vi "数据上传Z070A.vi"(1 "数据数组":string[](array[string]), 2 "合格Z030":bool, 3 "操作者":string, 4 "产品ID":string) -> ()   [LabVIEW 2011]
uses:
  <vilib>/Utility/error.llb/whitespace.ctl
panel:
  in  "error in (no error)":errorcluster
  out "error out":errorcluster
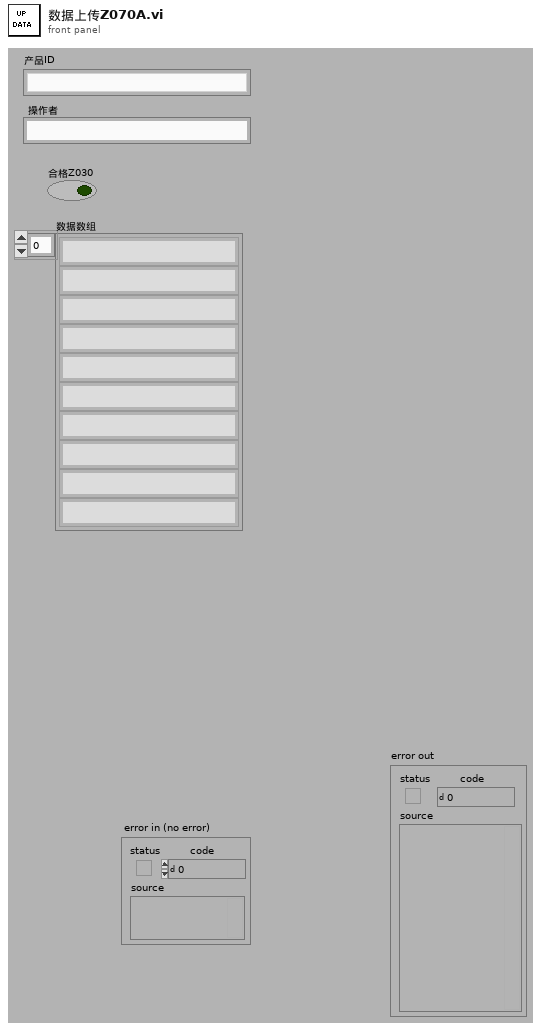
[diagram p1: front panel]
types:
  T1 = typedef "whitespace.ctl" = u16
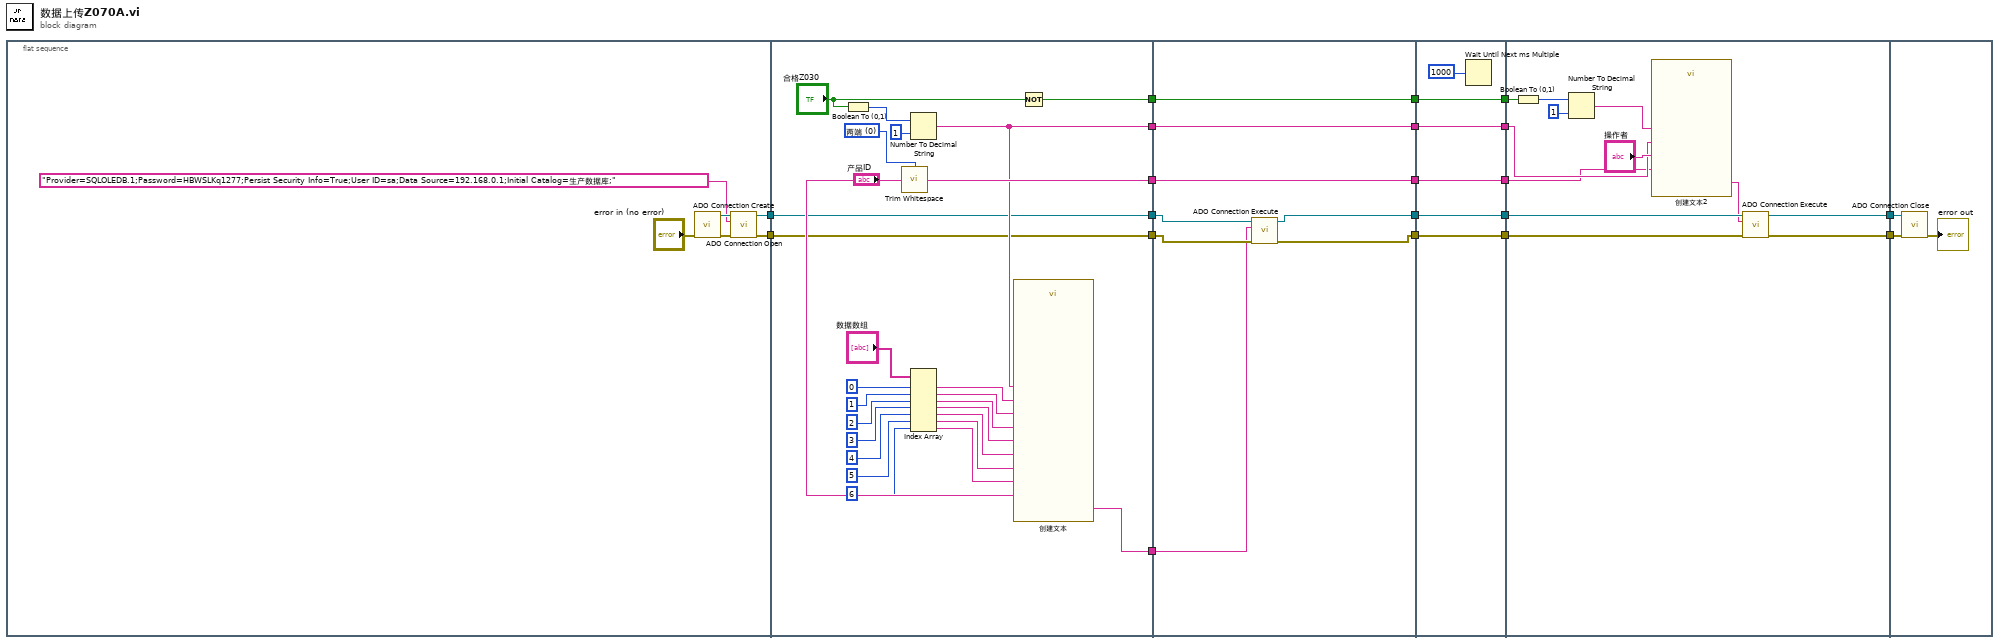
[diagram p0: block diagram]
diagram:
  n1 = flat-sequence {
    tunnel: [w22] -> w20
    tunnel: [w23] -> w19
    tunnel: w20 -> [w27]
    tunnel: w19 -> [w28]
    tunnel: [w28] -> w11
    tunnel: [w27] -> w9
    tunnel: [w43] -> w7
    tunnel: [w44] -> w5
    tunnel: [w46] -> w3
    tunnel: [w29] -> w1
    tunnel: w11 -> [w57]
    tunnel: [w56] -> w10
    tunnel: w9 -> [w55]
    tunnel: [w54] -> w8
    tunnel: w7 -> [w60]
    tunnel: [w60] -> w6
    tunnel: w5 -> [w59]
    tunnel: [w59] -> w4
    tunnel: w3 -> [w58]
    tunnel: [w58] -> w2
    tunnel: w1 -> [w53]
    tunnel: w10 -> [w66]
    tunnel: [w66] -> w18
    tunnel: w8 -> [w65]
    tunnel: [w65] -> w17
    tunnel: w6 -> [w64]
    tunnel: [w64] -> w16
    tunnel: w4 -> [w63]
    tunnel: [w63] -> w15
    tunnel: [w61] -> w12
    tunnel: w2 -> [w61]
    tunnel: w18 -> [w72]
    tunnel: w17 -> [w71]
    tunnel: w16 -> [w74]
    tunnel: w15 -> [w73]
    tunnel: [w69] -> w14
    tunnel: [w68] -> w13
    tunnel: w12 -> [w67]
    tunnel: w14 -> [w80]
    tunnel: w13 -> [w79]
    frame #0 {
      n2 = call "ADO Connection Create.vi"("error in (no error)"="error in (no error)") -> ("error out"=w25:errorcluster, "ADODB._Connection Out"=w24:refnum<k7>)  [unwired: 9 out]
      n3 = call "ADO Connection Open.vi"("error in (no error)"=w25, "ConnectionString"="Provider=SQLOLEDB.1;Password=HBWSLKq1277;Persist Security Info=True;User ID=sa;Data Source=192.168.0.1;Initial Catalog=生产数据库;" ("字符串 2"), "ADODB._Connection In"=w24) -> ("error out"=w22:errorcluster, "ADODB._Connection Out"=w23:refnum<k7>)  [unwired: 7 out]
    }
    frame #1 {
      w52 = T1 0 items=["两端", "字符串首端", "字符串末端"] ("location (both)")
      n4 = Boolean To (0,1)(Boolean="合格Z030") -> (0, 1=w51:i16)
      n5 = call <vilib>:"Trim Whitespace.vi"("string"="产品ID", "location (both)"=w52) -> ("trimmed string"=w44:string)
      n6 = Number To Decimal String(number=w51, width (-)=i16 1 ("宽度(-)")) -> (decimal integer string=w43:string)
      n7 = Index Array(array="数据数组", index #1=0 ("索引"), index #2=1 ("索引"), index #3=2 ("索引"), index #4=3 ("索引"), index #5=4 ("索引"), index #6=5 ("索引"), index #7=6 ("索引")) -> (element #1=w42:string, element #2=w41:string, element #3=w40:string, element #4=w39:string, element #5=w38:string, element #6=w37:string, element #7=w36:string)
      n8 = call "创建文本"("合格"=w43, "左空载峰值扭矩"=w42, "左空载平均扭矩"=w41, "左空载扭差"=w40, "右空载峰值扭矩"=w39, "右空载平均扭矩"=w38, "右空载扭差"=w37, "间隙值"=w36, "产品ID"=w44) -> ("Result"=w29:string)  [unwired: 17 in, 1 out]
      n9 = Not(x="合格Z030") -> (.not. x?=w46:bool)
    }
    frame #2 {
      n10 = call "ADO Connection Execute.vi"("error in (no error)"=w55, "CommandText"=w53, "ADODB._Connection In"=w57) -> ("error out"=w54:errorcluster, "ADODB._Connection Out"=w56:refnum<k7>)  [unwired: 7 out]
    }
    frame #3 {
      n11 = Wait Until Next ms Multiple(millisecond multiple=u32 1000 ("毫秒倍数")) -> ()  [unwired: 1 out]
    }
    frame #4 {
      n12 = Boolean To (0,1)(Boolean=w67) -> (0, 1=w75:i16)
      n13 = Number To Decimal String(number=w75, width (-)=i16 1 ("宽度(-)")) -> (decimal integer string=w77:string)
      n14 = call "创建文本2"("产品ID"=w73, "操作者"="操作者", "本序不合格"=w77, "本序合格"=w74) -> ("Result"=w70:string)  [unwired: 10 in, 1 out]
      n15 = call "ADO Connection Execute.vi"("error in (no error)"=w71, "CommandText"=w70, "ADODB._Connection In"=w72) -> ("error out"=w68:errorcluster, "ADODB._Connection Out"=w69:refnum<k7>)  [unwired: 7 out]
    }
    frame #5 {
      n16 = call "ADO Connection Close.vi"("error in (no error)"=w79, "ADODB._Connection In"=w80) -> ("error out"=→"error out":errorcluster)  [unwired: 9 out]
    }
  }
